vi "Constructor.vi"(8 "error in (no error)":errorcluster) -> (0 "error out":errorcluster, 2 "Keyboard":refnum<event-registration>, 3 "Keyboard out":refnum<class "Keyboard.lvclass">)   [LabVIEW 2021, in "InputDevice.lvlib" / "Keyboard.lvclass"]
uses:
  Keyboard.lvclass
  data.ctl
  Keyboard.lvclass/Keyboard.ctl
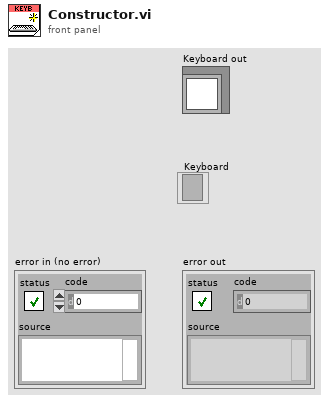
[diagram p1: front panel]
types:
  T1 = typedef "InputDevice.lvlib/Keyboard.lvclass/data.ctl" = cluster{"DeviceID":refnum<k1>, "Key Pressed":refnum<user-event>, "KeyPressedEvents":refnum<event-registration>, "StopNotifier":refnum<notifier>}
  T2 = enum16{"0", "1", "2", "3", "4", "5", "6", "7", "8", "9", "A", "B", "C", "D", "E", "F", "G", "H", "I", "J", "K", "L", "M", "N", "O", "P", "Q", "R", "S", "T", "U", "V", "W", "X", "Y", "Z", "F1", "F2", "F3", "F4", "F5", "F6", "F7", "F8", "F9", "F10", "F11", "F12", "F13", "F14", "F15", "ADD", "BACK", "BACKSLASH", "CAPITAL", "COMMA", "DECIMAL", "DELETE", "DIVIDE", "DOWN", "END", "EQUALS", "ESCAPE", "GRAVE (`)", "HOME", "INSERT", "LBRACKET", "LCONTROL", "LEFT", "L ALT", "LSHIFT", "LWIN", "MINUS", "MULTIPLY", "NEXT", "NUMLOCK", "NUMPAD_0", "NUMPAD_1", "NUMPAD_2", "NUMPAD_3", "NUMPAD_4", "NUMPAD_5", "NUMPAD_6", "NUMPAD_7", "NUMPAD_8", "NUMPAD_9", "PAUSE", "PERIOD", "PRIOR (PG UP)", "RBRACKET", "RCONTROL", "RETURN", "RIGHT", "R ALT", "RSHIFT", "RWIN", "SCROLL", "SEMICOLON", "SLASH", "SPACE", "SUBTRACT", "TAB", "UP", "ENTER (num pad)", "' (quote)"}[]
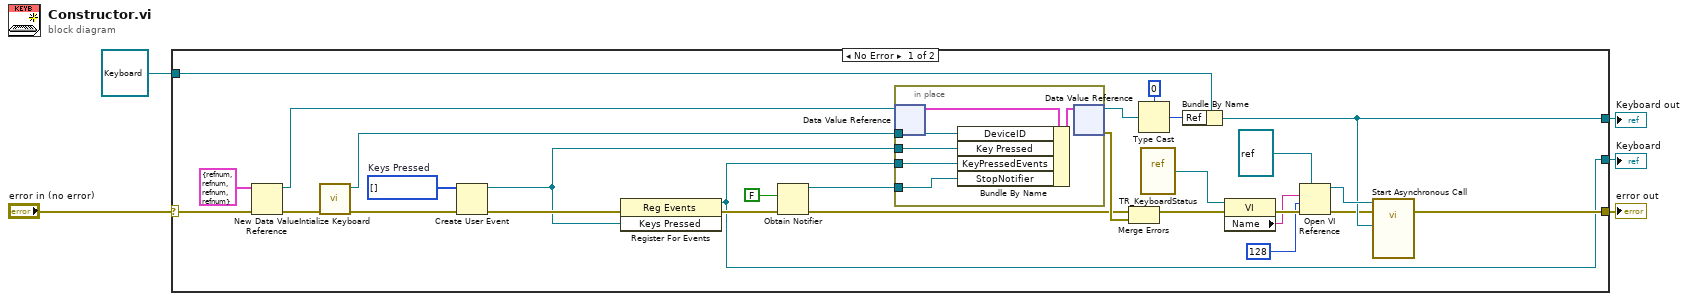
[diagram p0: block diagram]
diagram:
  n1 = case shown="No Error" "error in (no error)" {
    selector: "error in (no error)" -> [w28 w42]
    tunnel: [w10 w42] -> w4
    tunnel: [w12 w41] -> w3
    tunnel: refnum<class "Keyboard.lvclass"> refnum ("Keyboard out") -> [w32 w41]
    tunnel: [w7 _] -> w1
    frame No Error {
      w8 = T2 [] items=["0", "1", "2", "3", "4", "5", "6", "7", "8", "9", "A", "B", "C", "D", "E", "F", "G", "H", "I", "J", "K", "L", "M", "N", "O", "P", "Q", "R", "S", "T", "U", "V", "W", "X", "Y", "Z", "F1", "F2", "F3", "F4", "F5", "F6", "F7", "F8", "F9", "F10", "F11", "F12", "F13", "F14", "F15", "ADD", "BACK", "BACKSLASH", "CAPITAL", "COMMA", "DECIMAL", "DELETE", "DIVIDE", "DOWN", "END", "EQUALS", "ESCAPE", "GRAVE (`)", "HOME", "INSERT", "LBRACKET", "LCONTROL", "LEFT", "L ALT", "LSHIFT", "LWIN", "MINUS", "MULTIPLY", "NEXT", "NUMLOCK", "NUMPAD_0", "NUMPAD_1", "NUMPAD_2", "NUMPAD_3", "NUMPAD_4", "NUMPAD_5", "NUMPAD_6", "NUMPAD_7", "NUMPAD_8", "NUMPAD_9", "PAUSE", "PERIOD", "PRIOR (PG UP)", "RBRACKET", "RCONTROL", "RETURN", "RIGHT", "R ALT", "RSHIFT", "RWIN", "SCROLL", "SEMICOLON", "SLASH", "SPACE", "SUBTRACT", "TAB", "UP", "ENTER (num pad)", "' (quote)"]  # Keys Pressed
      n2 = New Data Value Reference(data value=T1 {"DeviceID"=refnum, "Key Pressed"=refnum, "KeyPressedEvents"=refnum, "StopNotifier"=refnum} ("Cluster"), error in=w28) -> (data value reference=w33:refnum<data-value>, error out=w27:errorcluster)
      n3 = call <vilib>:"Intialize Keyboard.vi"("error in (no error)"=w27) -> ("error out"=w24:errorcluster, "device ID"=w26:refnum<k1>)  [unwired: 9 in]
      n4 = Create User Event(user event datatype=w8, error in=w24) -> (user event=w6:refnum<user-event>, error out=w23:errorcluster)
      n5 = register-events(error in=w23, w6) -> (reference out=w7:refnum<event-registration>, error out=w21:errorcluster)  [unwired: 1 in]
      n6 = Obtain Notifier(notification data type=FALSE, error in (no error)=w21) -> (notifier out=w9:refnum<notifier>, error out=w20:errorcluster)  [unwired: 2 in, 1 out]
      n7 = in-place {
        in-place-border: w26 -> [w38]
        in-place-border: w6 -> [w37]
        in-place-border: w7 -> [w35]
        in-place-border: w9 -> [w36]
        n8 = in-place-dvr #1(w33) -> (w40:T1)  [unwired: 1 out]
        n9 = Bundle By Name(cluster=w40, "DeviceID"=w38, "Key Pressed"=w37, "KeyPressedEvents"=w35, "StopNotifier"=w36) -> (w39:T1)
        n10 = in-place-dvr #1(w39) -> (w31:refnum<data-value>, w25:errorcluster)
      }
      n11 = Merge Errors(w20, w25) -> (w19:errorcluster)
      n12 = Type Cast(type=u64 0 ("Ref"), x=w31) -> (*(type *) &x=w29:u64)
      n13 = vi-ref "TR_KeyboardStatus.vi"() -> (w15:refnum<vi>)
      n14 = Bundle By Name(cluster=w32, "Ref"=w29) -> (w12:refnum<class "Keyboard.lvclass">)
      n15 = property class="VI"(reference=w15, error in=w19) -> (error out=w18:errorcluster, "Name"=w17:string)  [unwired: 1 out]
      n16 = Open VI Reference(type specifier VI Refnum (for type only)=refnum<vi> refnum, vi path=w17, options=128, error in (no error)=w18) -> (vi reference=w14:refnum<vi>, error out=w11:errorcluster)  [unwired: 2 in]
      n17 = call-by-ref "Start Asynchronous Call"(reference=w14, error in=w11, "Mouse in"=w12) -> (error out=w10:errorcluster)  [unwired: 11 in, 1 out]
    }
    frame Error {
    }
  }
  "error out" <- w4
  "Keyboard out" <- w3
  "Keyboard" <- w1
